vi "S2C_OM8257_Proc_Globals.vi"() -> ()   [LabVIEW 2015]
panel:
  in  "8257-Visa":refnum<visa-resource-name>
  out "8257-Refs":string[][](array[string])
  in  "8257-VI":refnum<vi>
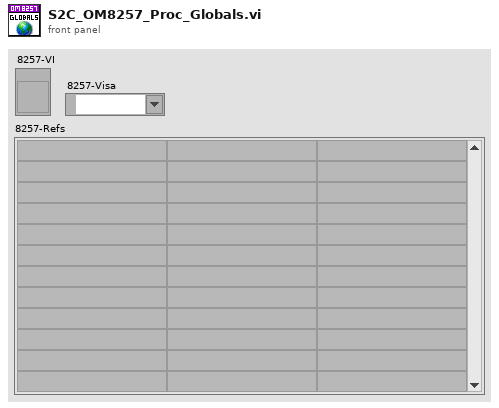
[diagram p1: front panel]
diagram:
